vi "HDF5_array_mod_Zoom.vi"(10 "delta":dbl, 11 "Array in":T1[][](array[typedef])) -> (3 "Array out":T1[][](array[typedef]))   [LabVIEW 2018]
uses:
  HDF5/HDF5_ToneInfoZoomAryClust.ctl
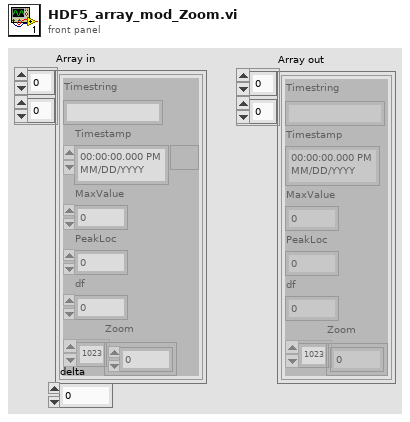
[diagram p1: front panel]
types:
  T1 = typedef "HDF5_ToneInfoZoomAryClust.ctl" = cluster{"Timestring":string, "Timestamp":timestamp, "MaxValue":dbl, "PeakLoc":dbl, "df":dbl, "Zoom":dbl[]}
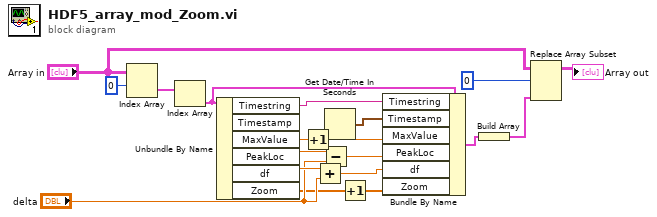
[diagram p0: block diagram]
diagram:
  n1 = Index Array(array="Array in", index (row)=0) -> (element=w18:T1[])  [unwired: 1 in]
  n2 = Index Array(array=w18) -> (element=w7:T1)  [unwired: 1 in]
  n3 = Unbundle By Name(w7) -> ("Timestring"=w8:string, "MaxValue"=w13:dbl, "PeakLoc"=w14:dbl, "df"=w15:dbl, "Zoom"=w2:dbl[])  [unwired: 1 out]
  n4 = Increment(x=w13) -> (x+1=w11:dbl)
  n5 = Add(x=w15, y="delta") -> (x+y=w12:dbl)
  n6 = Subtract(x=w14, y="delta") -> (x-y=w10:dbl)
  n7 = Get Date/Time In Seconds() -> (seconds since 1Jan1904=w9:timestamp)
  n8 = Increment(x=w2) -> (x+1=w1:dbl[])
  n9 = Bundle By Name(cluster=w7, "Timestring"=w8, "Timestamp"=w9, "MaxValue"=w11, "PeakLoc"=w10, "df"=w12, "Zoom"=w1) -> (w6:T1)
  n10 = Build Array(w6) -> (w4:T1[])
  n11 = Replace Array Subset(array="Array in", new element=w4, index (row)=0) -> (→"Array out":T1[][])  [unwired: 1 in]
